vi "Setup Timer.vi"(5 "Enqueue Next State":bool, 6 "Timer ID":i32, 7 "Next State":string, 8 "error in (no error)":errorcluster, 9 "Count":i32, 10 "Period":i32, 11 "Timer On":bool) -> (0 "error out":errorcluster)   [LabVIEW 2015, in "Tool Module.lvlib"]
doc: "<b>Note</b>: This VI was renamed by the DQMH Rename Event utility. Make sure the VI Description is updated to reflect the new event name, then delete this comment.\n\nStart/Stop and specify the timing period and number of time periods (Count) for Timer 1.\n_____\nCreated using Delacor QMH Event Scripter 4.2.1.88."
uses:
  Tool Module.lvlib
  Setup Timer Argument--cluster.ctl
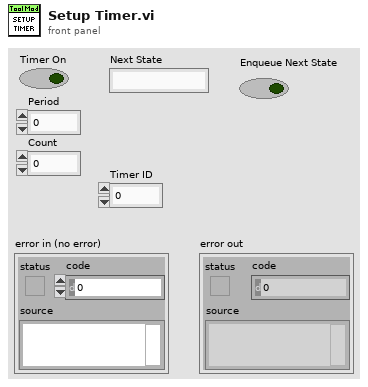
[diagram p1: front panel]
types:
  T1 = typedef "Tool Module.lvlib/Setup Timer Argument--cluster.ctl" = cluster{"Timer ID":i32, "Timer On":bool, "Period":i32, "Count":i32, "Next State":string, "Enqueue Next State":bool}
  T2 = typedef "Tool Module.lvlib/Request Events--cluster.ctl" = cluster{"Stop Module":refnum<user-event>, "Show Panel":refnum<user-event>, "Hide Panel":refnum<user-event>, "Get Module Execution Status":refnum<user-event>, "Show Diagram":refnum<user-event>, "GOTO":refnum<user-event>, "CONNECT":refnum<user-event>, "Get All Inspect Data":refnum<user-event>, "Start Data Monitor":refnum<user-event>, "Get FPGA Setup Params":refnum<user-event>, "Set FPGA Setup Params":refnum<user-event>, "Commit Tool Config":refnum<user-event>, "Set Integration Count":refnum<user-event>, "Set Laser Params":refnum<user-event>, "Get Mtrl Ctrl Reg":refnum<user-event>, "Commit Ctrl Reg":refnum<user-event>, "Set Event Logger":refnum<user-event>, "Write to File":refnum<user-event>, "Read from File":refnum<user-event>, "Set Device Temp Thresholds":refnum<user-event>, "Get Cycle Count":refnum<user-event>, "Return FPGA Setup Data":refnum<user-event>, "Update FPGA Setup Data":refnum<user-event>, "Setup Timer":refnum<user-event>, "Tool Status Reader Cmd":refnum<user-event>, "Stop Helper Loops":refnum<user-event>, "Enable Receive Stream":refnum<user-event>, "Get-Set Inspection Limits":refnum<user-event>, "INSPECT":refnum<user-event>}
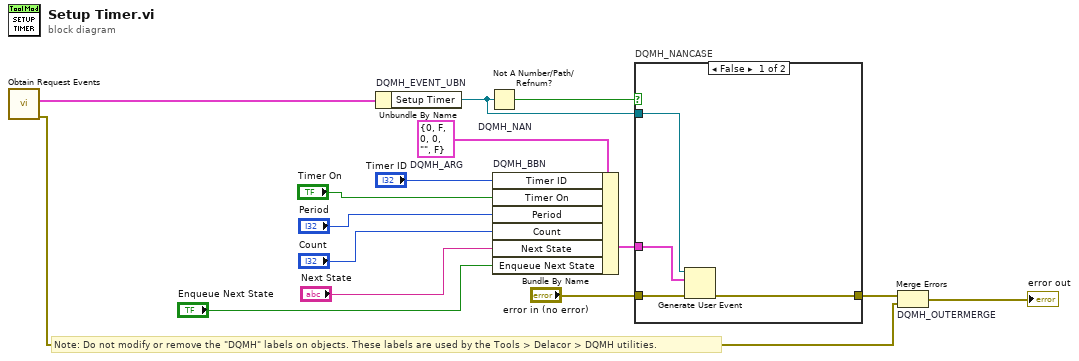
[diagram p0: block diagram]
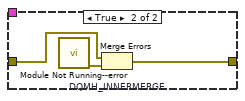
[diagram p2: hidden frame]
diagram:
  w9 = T1 {"Timer ID"=0, "Timer On"=FALSE, "Period"=0, "Count"=0, "Next State"="", "Enqueue Next State"=FALSE}  # DQMH_ARG
  # "Note: Do not modify or remove the \"DQMH\" labels on objects. These labels are used by the Tools > Delacor > DQMH utilities."
  n1 = call "Obtain Request Events.vi"() -> ("error out"=w8:errorcluster, "Tool Module Request Events"=w7:T2)  [unwired: 10 in]
  n2 = Unbundle By Name "DQMH_EVENT_UBN"(w7) -> ("Setup Timer"=w11:refnum<user-event>)
  n3 = Not A Number/Path/Refnum? "DQMH_NAN"(number/path/refnum=w11) -> (NaN/Path/Refnum?=w12:bool)
  n4 = Bundle By Name "DQMH_BBN"(cluster=w9, "Timer ID"="Timer ID", "Timer On"="Timer On", "Period"="Period", "Count"="Count", "Next State"="Next State", "Enqueue Next State"="Enqueue Next State") -> (w13:T1)
  n5 = case "DQMH_NANCASE" shown="False" w12 {
    tunnel: "error in (no error)" -> [w19 w22]
    tunnel: [w18 w21] -> w10
    tunnel: w11 -> [w17 _]
    tunnel: w13 -> [w16 _]
    frame False {
      n6 = Generate User Event(user event=w17, event data cluster=w16, error in=w19) -> (error out=w18:errorcluster)  [unwired: 1 in, 1 out]
    }
    frame True {
      n7 = call "Module Not Running--error.vi"() -> ("error out"=w20:errorcluster)  [unwired: 11 in]
      n8 = Merge Errors "DQMH_INNERMERGE"(w22, w20) -> (w21:errorcluster)
    }
  }
  n9 = Merge Errors "DQMH_OUTERMERGE"(w10, w8) -> (→"error out":errorcluster)
